vi "Running.vi"(8 "error in (no error)":errorcluster, 11 "CIFTemplatePlugin in":refnum<class "TemplatePlugin.lvclass">) -> (0 "error out":errorcluster, 2 "Destroy":bool, 3 "CIFTemplatePlugin out":refnum<class "TemplatePlugin.lvclass">)   [LabVIEW 2021, in "TemplatePlugin.lvclass"]
uses:
  TemplatePlugin.lvclass
  D:/dev/CIF-LVCore/src/CIFCore/Class/CIFCorePlugin.lvclass
  CIF-LVCore/src/CIFCore/Class/CIFCorePlugin.lvclass/CIFCorePlugin.ctl
  TemplatePlugin.lvclass/TemplatePlugin.ctl
  <vilib>/CIF Foundation/CIF Utilities/Statistics/I64/Stats_I64_CIF_U.lvclass/Stats_I64_CIF_U.ctl
  CIF-LVCore/src/Channels/CIFChannelMng/CIFChannelMng.lvclass/CIFChannelMng.ctl
  <vilib>/CIF Foundation/CIF Channels Core/CIFChannels/CIFChannels.lvclass/CIFChannels.ctl
  CIF-LVCore/src/CIFCore/Class/Typedef/Energized States.ctl
  Logic.vi
  CIF-LVCore/src/CIFCore/Class/Accessors/Write Energized State.vi
  CIF-LVCore/src/CIFCore/Class/SubVIs/Sleep.vi
  CIF-LVCore/src/CIFCore/Class/SubVIs/OOB/Read Core OOB RX.vi
  OOB Comm/Read Comm to Main.vi
  OOB Comm/Send Cyclic to gRPC.vi
  CIF-LVCore/src/CIFCore/Class/SubVIs/OOB/Update Status from Benchmarks.vi
  CIF-LVCore/src/Channels/CIFChannelMng/Core/Send Channel List Update.vi
  CIF-LVCore/src/CIFCore/Class/SubVIs/OOB/Send Core OOB TX.vi/074d8088-3ad4-4fdc-9542-b009f1b06b72.vi
  <vilib>/CIF Foundation/CIF Utilities/Time/System Time/Sleep Until Future Time.vi
  <vilib>/CIF Foundation/CIF Utilities/Time/System Time/Get System Time.vi
  CIF-LVCore/src/CIFCore/Class/Channel RW/Read U64.vi
  CIF-LVCore/src/CIFCore/Class/Channel RW/Write U64.vi
  CIF-LVCore/src/CIFCore/Class/Channel RW/Write Double.vi
  CIF-LVCore/src/CIFCore/Class/Channel RW/Read Double.vi
  CIF-LVCore/src/CIFCore/Class/Accessors/Monitor/Write Double 1.vi
  CIF-LVCore/src/CIFCore/Class/Accessors/Monitor/Write U64 1.vi
  CIF-LVCore/src/CIFCore/Class/Accessors/Monitor/Write U64 2.vi
  CIF-LVCore/src/CIFCore/Class/Accessors/Monitor/Write I64 1.vi
  CIF-LVCore/src/CIFCore/Class/Accessors/Monitor/Write I64 2.vi
  CIF-LVCore/src/CIFCore/Class/Accessors/Timestamps/Write Execute TS.vi
  CIF-LVCore/src/CIFCore/Class/Accessors/Timestamps/Write Sleep TS.vi
  <vilib>/Utility/error.llb/Clear Errors.vi
  CIF-LVCore/src/CIFCore/Class/Accessors/Read Sleep Limits (ns).vi
  CIF-LVCore/src/CIFCore/Class/Accessors/Timestamps/Write Target Wake TS.vi
  CIF-LVCore/src/CIFCore/Class/Accessors/Read Plugin Name.vi
  CIF-LVCore/src/CIFCore/Common/Utilities/Add Error.vi
  CIF-LVCore/src/CIFCore/Class/Accessors/Timestamps/Read Running TS.vi
  CIF-LVCore/src/CIFCore/Class/Benchmarking/Reset Delay.vi
  CIF-LVCore/src/CIFCore/Class/Accessors/Read Running Internal Data.vi
  CIF-LVCore/src/CIFCore/Class/Accessors/Read Timing Override.vi
  CIF-LVCore/src/CIFCore/Class/Accessors/Read Common Config.vi
  CIF-LVCore/src/CIFCore/Class/Accessors/Timestamps/Write Housekeeping TS.vi
  <vilib>/CIF Foundation/CIF Utilities/Statistics/I64/X1 minus X0.vi
  <vilib>/CIF Foundation/CIF Utilities/Statistics/I64/Cyclic.vi
  CIF-LVCore/src/CIFCore/Class/Accessors/Timestamps/Read Execute TS.vi
  CIF-LVCore/src/CIFCore/Class/Accessors/Timestamps/Read Housekeeping TS.vi
  CIF-LVCore/src/CIFCore/Class/Accessors/Timestamps/Read Sleep TS.vi
  CIF-LVCore/src/CIFCore/Class/Accessors/Timestamps/Read Target Wake TS.vi
  CIF-LVCore/src/CIFCore/Class/SubVIs/Refresh Stats.vi
  CIF-LVCore/src/CIFCore/Class/SubVIs/OOB/Receive/Read Clock Map.vi
  CIF-LVCore/src/CIFCore/Class/SubVIs/OOB/Receive/Read Connections.vi
  CIF-LVCore/src/Channels/CIFChannelMng/SubVIs/Connect Channel.vi
  CIF-LVCore/src/CIFCore/Class/SubVIs/OOB/Receive/Read Forces.vi
  CIF-LVCore/src/Channels/CIFChannelMng/SubVIs/Force Channel.vi
  CIF-LVCore/src/Channels/CIFChannelMng/SubVIs/Add FIFO Publisher.vi
  CIF-LVCore/src/CIFCore/Class/SubVIs/OOB/Receive/Read Publisher Instance.vi
  CIF-LVCore/src/Channels/CIFChannelMng/Core/Send Publisher Instance Return.vi
  CIF-LVCore/src/Channels/CIFChannelMng/SubVIs/Remove FIFO Publisher.vi
  CIF-LVCore/src/CIFCore/Class/SubVIs/OOB/Read Core OOB RX.vi/a31a91a9-4107-4750-8e0d-44486e9a3a34.vi
  OOB Comm/Read Comm to Main.vi/525c214c-2a6b-4e7b-b3ce-0ad96b412d2f.vi
  OOB Comm/Read Comm to Main.vi/4efb0375-f1de-4191-b03f-44d34e6646cb.vi
  OOB Comm/Send Cyclic to gRPC.vi/0c0f428d-7269-422d-ba27-f9d6fa7232ec.vi
  CIF-LVCore/src/CIFCore/Class/Accessors/Read Refresh.vi
  <vilib>/CIF Foundation/CIF Utilities/Statistics/I64/Get Stats.vi
  CIF-LVCore/src/Channels/CIFChannelMng/Core/Send Channel List Update.vi/463ebf4c-8748-40f9-8ad3-9e61c16a01a6.vi
  <vilib>/CIF Foundation/CIF CIPC/SubVIs/Check Error.vi
  <vilib>/CIF Foundation/CIF CIPC/SubVIs/Notify Of New Write.vi
  <vilib>/CIF Foundation/CIF CIPC/SubVIs/Get dll Path.vi
  <vilib>/CIF Foundation/CIF CIPC/SubVIs/Get Element Write Position.vi
  <vilib>/CIF Foundation/CIF Utilities/Time/SubVIs/Add Error.vi
  <vilib>/CIF Foundation/CIF Utilities/Time/System Time/LabVIEW Time to TAI Time.vi
  <vilib>/CIF Foundation/CIF Utilities/Errors/Append Error Location.vi
  <vilib>/CIF Foundation/CIF Utilities/Statistics/I64/X1 minus X0.vi/dfabcf33-0dbc-4041-80a5-3dc0c86d2989.vi
  <vilib>/CIF Foundation/CIF Utilities/Statistics/I64/Cyclic.vi/dfabcf33-0dbc-4041-80a5-3dc0c86d2989.vi
  CIF-LVCore/src/Channels/CIFChannelMng/Utilities/Get Channel Index by Name.vi
  <vilib>/CIF Foundation/CIF Channels Core/CIFChannels/Accessors/Read Channel State.vi
  <vilib>/CIF Foundation/CIF Channels Core/CIFChannels/Accessors/Read Tag Forced.vi
  CIF-LVCore/src/Channels/CIFChannelMng/SubVIs/Add Error Channel Manager.vi
  CIF-LVCore/src/Channels/CIFChannelMng/Core/Send Publisher Instance Return.vi/9db40550-ae0b-4108-a32d-02e81b824dbe.vi
  CIF-LVCore/src/Channels/CIFChannelMng/SubVIs/Get Original FIFO Channel Name.vi
  <vilib>/CIF Foundation/CIF CIPC/SubVIs/Wait For N Elements Available.vi
  <vilib>/CIF Foundation/CIF CIPC/SubVIs/Get Element Read Position.vi
  <vilib>/CIF Foundation/CIF CIPC/SubVIs/Set Element Read Position.vi
  <vilib>/CIF Foundation/CIF Utilities/Statistics/I64/X1 minus X0.vi/dfabcf33-0dbc-4041-80a5-3dc0c86d2989.vi/9eb60a9a-770f-4d2d-8b3f-8465c267ecc9.vi
  <vilib>/CIF Foundation/CIF Utilities/Statistics/I64/Cyclic.vi/dfabcf33-0dbc-4041-80a5-3dc0c86d2989.vi/9eb60a9a-770f-4d2d-8b3f-8465c267ecc9.vi
  <vilib>/CIF Foundation/CIF Channels Core/ChannelCommon/Utilities/Add Error.vi
  <vilib>/CIF Foundation/CIF CIPC/SubVIs/Get Element Info Variant.vi
  <vilib>/Utility/error.llb/Trim Whitespace.vi
  <vilib>/Utility/error.llb/Error Cluster From Error Code.vi
  <vilib>/CIF Foundation/CIF Channels Core/CIFChannels/Core/Set Force.vi
  <vilib>/CIF Foundation/CIF Channels Core/CIFChannels/CIFChannels.lvclass
  CIF-LVCore/src/CIFCore/Class/CIFCorePlugin.lvclass
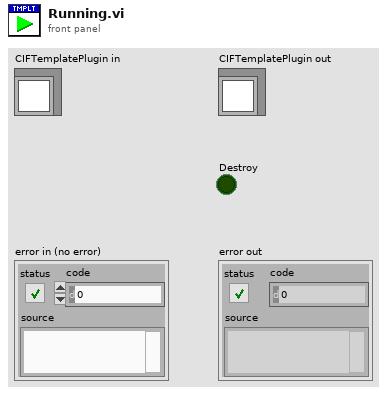
[diagram p1: front panel]
types:
  T1 = typedef "CIFCorePlugin.lvclass/Energized States.ctl" = enum16{"Listen", "Prepare", "Execute", "Housekeep", "Cleanup", "Destroy"}
  T2 = typedef "CIFCorePlugin.lvclass/Running State Logic.ctl" = enum16{"Execute", "Housekeep", "Cleanup", "Error", "Destroy"}
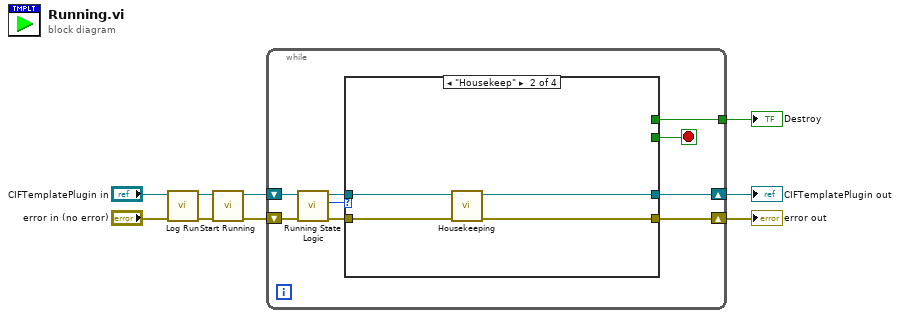
[diagram p0: block diagram]
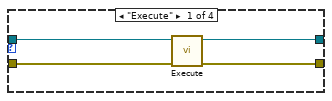
[diagram p2: hidden frame]
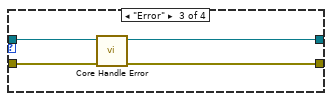
[diagram p3: hidden frame]
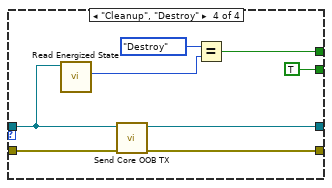
[diagram p4: hidden frame]
diagram:
  n1 = call "Log Run.vi"("error in (no error)"="error in (no error)", "CIFCorePlugin in"="CIFTemplatePlugin in") -> ("error out"=w7:errorcluster, "CIFCorePlugin out"=w6:refnum<class "TemplatePlugin.lvclass">)  [unwired: 8 in]
  n2 = call "Start Running.vi"("error in (no error)"=w7, "CIFCorePlugin in"=w6) -> ("error out"=w8:errorcluster, "CIFCorePlugin out"=w9:refnum<class "TemplatePlugin.lvclass">)  [unwired: 8 in]
  n3 = while {
    shift-right: [w13] -> w4
    shift-left: w9 -> [w18]
    shift-right: [w12] -> w3
    shift-left: w8 -> [w17]
    tunnel: [w10] -> w5
    stop <- w11 stop-if-true
    n4 = call "Running State Logic.vi"("error in (no error)"=w17, "CIFCorePlugin in"=w18) -> ("error out"=w14:errorcluster, "Running State Logic"=w16:T2, "CIFCorePlugin out"=w15:refnum<class "TemplatePlugin.lvclass">)  [unwired: 7 in]
    n5 = case shown="\"Housekeep\"" w16 {
      tunnel: w15 -> [w22 w26 w30 w32]
      tunnel: w14 -> [w21 w25 w29 w37]
      tunnel: [w20 w24 w28 w36] -> w13
      tunnel: [w19 w23 w27 w35] -> w12
      tunnel: [_ _ _ TRUE] -> w11
      tunnel: [_ _ _ w33] -> w10
      frame "Execute" {
        n6 = call "Execute.vi"("error in (no error)"=w21, "CIFTemplatePlugin in"=w22) -> ("error out"=w19:errorcluster, "CIFTemplatePlugin out"=w20:refnum<class "TemplatePlugin.lvclass">)  [unwired: 8 in]
      }
      frame "Housekeep" {
        n7 = call "Housekeeping.vi"("error in (no error)"=w25, "CIFTemplatePlugin in"=w26) -> ("error out"=w23:errorcluster, "CIFTemplatePlugin out"=w24:refnum<class "TemplatePlugin.lvclass">)  [unwired: 8 in]
      }
      frame "Error" {
        n8 = call "Core Handle Error.vi"("error in (no error)"=w29, "CIFTemplateNode in"=w30) -> ("error out"=w27:errorcluster, "CIFTemplateNode out"=w28:refnum<class "TemplatePlugin.lvclass">)  [unwired: 8 in]
      }
      frame "Cleanup", "Destroy" {
        n9 = call "Read Energized State.vi"("CIFCorePlugin in"=w32) -> ("Energized State"=w31:T1)  [unwired: 8 in, 2 out]
        n10 = call "Send Core OOB TX.vi"("error in (no error)"=w37, "CIFCorePlugin in"=w32) -> ("error out"=w35:errorcluster, "CIFCorePlugin out"=w36:refnum<class "TemplatePlugin.lvclass">)  [unwired: 8 in]
        n11 = Equal?(x=Energized_States."Destroy", y=w31) -> (x = y?=w33:bool)
      }
    }
  }
  "error out" <- w3
  "Destroy" <- w5
  "CIFTemplatePlugin out" <- w4
